vi "XY Sub_VI.vi"(3 "error in (no error)":errorcluster, 5 "XY Cluster In":T1 {"Y Data"."Input"."Tol" min=0.0; "X Data"."Input"."Tol" min=0.0}) -> (0 "error out":errorcluster, 2 "XY Cluster Out":T1={"X Data"={"Complete?"=FALSE, "Motor Params"={"Duty %"=0.0, "X Freq"=0.0, "FWD/RVS"=FALSE}, "SP"={"Accel"=0.0, "Decel"=0.0, "Speed"=0.0}, "State"=enum."Stop", "Input"={"Coord"=0.0, "Tol"=0.0, "Accel"=0.0, "Decel"=0.0, "Max Speed"=0.0}, "Path"={"V plan"=[], "V actual"=[], "S actual"=[], "a actual"=[], "Profile"=enum."Triangular", "Decel Dist"=0.0, "Accel Dist"=0.0, "Cruise V"=0.0, "Cruise Dist"=0.0}, "PID"={"Kc"=0.0, "Ti"=0.0, "Td"=0.0}, "Motion"={"Speed"=0.0, "Dist"=0.0, "Acceleration"=0.0, "Dist to target"=0.0}}, "Y Data"={"Complete?"=FALSE, "Motor Params"={"Duty %"=0.0, "Freq"=0.0, "FWD/RVS"=FALSE}, "SP"={"Y Accel"=0.0, "Y Decel"=0.0, "Speed"=0.0}, "State"=enum."Stop", "Input"={"Coord"=0.0, "Tol"=0.0, "Accel"=0.0, "Decel"=0.0, "Max Speed"=0.0}, "Path"={"V plan"=[], "V actual"=[], "S actual"=[], "a actual"=[], " Profile"=enum."Triangular", "Decel Dist"=0.0, "Accel Dist"=0.0, "Cruise V"=0.0, "Cruise Dist"=0.0}, "PID"={"Kc"=0.0, "Ti"=0.0, "Td"=0.0}, "Motion"={"Speed"=0.0, "Dist"=0.0, "Acceleration"=0.0, "Dist to target"=0.0}}, "Timing"={"Runtime"=0.0, "Loop time"=0.0, "Loop iter"=0, "Tick"=0.0}, "stop"=FALSE} {"Y Data"."Input"."Tol" min=0.0; "X Data"."Input"."Tol" min=0.0})   [LabVIEW 2017]
uses:
  Encoder Cluster.ctl
  <vilib>/myRIO/Common/Instrument Driver Framework/myRIO v1.0/Encoder/typedefs/Encoder Count Direction Enum.ctl
  XY Cluster.ctl
  Motor Status Enum.ctl
  Motion Type Def.ctl
  <vilib>/myRIO/Instrument Drivers/Onboard IO/PWM/typedefs/PWM Reference.ctl
  <vilib>/myRIO/Common/Instrument Driver Framework/Utilities/typedefs/myRIO Generic Hardware Reference.ctl
  <vilib>/myRIO/Common/Instrument Driver Framework/Utilities/typedefs/Hardware Version Enum.ctl
  <vilib>/myRIO/Common/Instrument Driver Framework/Utilities/typedefs/myRIO v1.0 Reference.ctl
  <vilib>/myRIO/Common/Instrument Driver Framework/Utilities/typedefs/Generic FPGA Reference.ctl
  <vilib>/myRIO/Common/Instrument Driver Framework/myRIO v1.0/PWM/typedefs/PWM Channels Enum.ctl
  <vilib>/myRIO/Instrument Drivers/Onboard IO/PWM/typedefs/PWM Configuration.ctl
  <vilib>/userdefined/High Color/nirio_resource_hc.ctl
  <vilib>/myRIO/Common/Instrument Driver Framework/Utilities/vis/Is FPGA Ref Available.vi
  <vilib>/myRIO/Common/Instrument Driver Framework/myRIO v1.0/PWM/vis/myRIO v1.1 Open PWM.vi
  <vilib>/myRIO/Instrument Drivers/Onboard IO/PWM/vis/Set Duty Cycle and Frequency.vi
  <vilib>/myRIO/Common/Instrument Driver Framework/Utilities/vis/Validate Channels.vi
  <vilib>/myRIO/Common/Instrument Driver Framework/myRIO v1.0/PWM/vis/myRIO v1.0 Reserve PWM.vi
  <vilib>/myRIO/Common/Instrument Driver Framework/myRIO v1.0/PWM/vis/myRIO v1.0 Build MUX Configuration PWM.vi
  <vilib>/myRIO/Common/Instrument Driver Framework/myRIO v1.0/Resource Manager/vis/myRIO v1.0 Reserve Channel List.vi
  <vilib>/myRIO/Common/Instrument Driver Framework/myRIO v1.0/Resource Manager/vis/myRIO v1.0 Create Configuration List.vi
  <vilib>/myRIO/Common/Instrument Driver Framework/myRIO v1.0/Resource Manager/vis/myRIO v1.0 Reserve Channel.vi
  <vilib>/myRIO/Common/Instrument Driver Framework/myRIO v1.0/Resource Manager/vis/myRIO v1.0 Unreserve Channel.vi
  <vilib>/myRIO/Common/Instrument Driver Framework/myRIO v1.0/Resource Manager/vis/myRIO v1.0 Build Mutex Name.vi
  <vilib>/addons/control/pid/pid.llb/PID Control Input Filter (DBL).vi
  <vilib>/addons/control/pid/pid.llb/PID (DBL).vi
  <vilib>/Utility/VariantDataType/GetNumericInfo.vi
  <vilib>/Utility/error.llb/Error Cluster From Error Code.vi
  <vilib>/myRIO/Common/Instrument Driver Framework/myRIO v1.0/myRIO v1.1 Open.vi
  <vilib>/myRIO/Common/Instrument Driver Framework/Utilities/vis/IO Manager.vi
  <vilib>/myRIO/Common/Instrument Driver Framework/Utilities/vis/Configuration Manager.vi
  <vilib>/myRIO/Common/Instrument Driver Framework/myRIO v1.0/Resource Manager/vis/myRIO v1.0 Configure IO.vi
  <vilib>/myRIO/Common/Instrument Driver Framework/myRIO v1.0/myRIO v1.0 Close.vi
  <vilib>/myRIO/Common/Instrument Driver Framework/myRIO v1.0/PWM/vis/myRIO v1.0 Write PWM.vi
  <vilib>/myRIO/Express VI/Onboard IO/PWM/PWM Express VI.xnode
  <vilib>/myRIO/Instrument Drivers/Onboard IO/PWM/vis/myRIO PWM Open.xnode
  <vilib>/addons/control/pid/NI_PID_pid.lvlib
  <vilib>/ptbypt/NI_PtbyPt.lvlib
  <vilib>/myRIO/Instrument Drivers/Onboard IO/PWM/PWM.lvlib
panel:
  out "Y PID":cluster{"mean":dbl, "output":dbl}(graph)
  out "X PID":cluster{"Speed":dbl, "output":dbl}(graph)
  out "Y dist > +20":bool
  out "X dist > +20":bool
  out "Encoder Output":T4
  out "X&Y Complete":bool
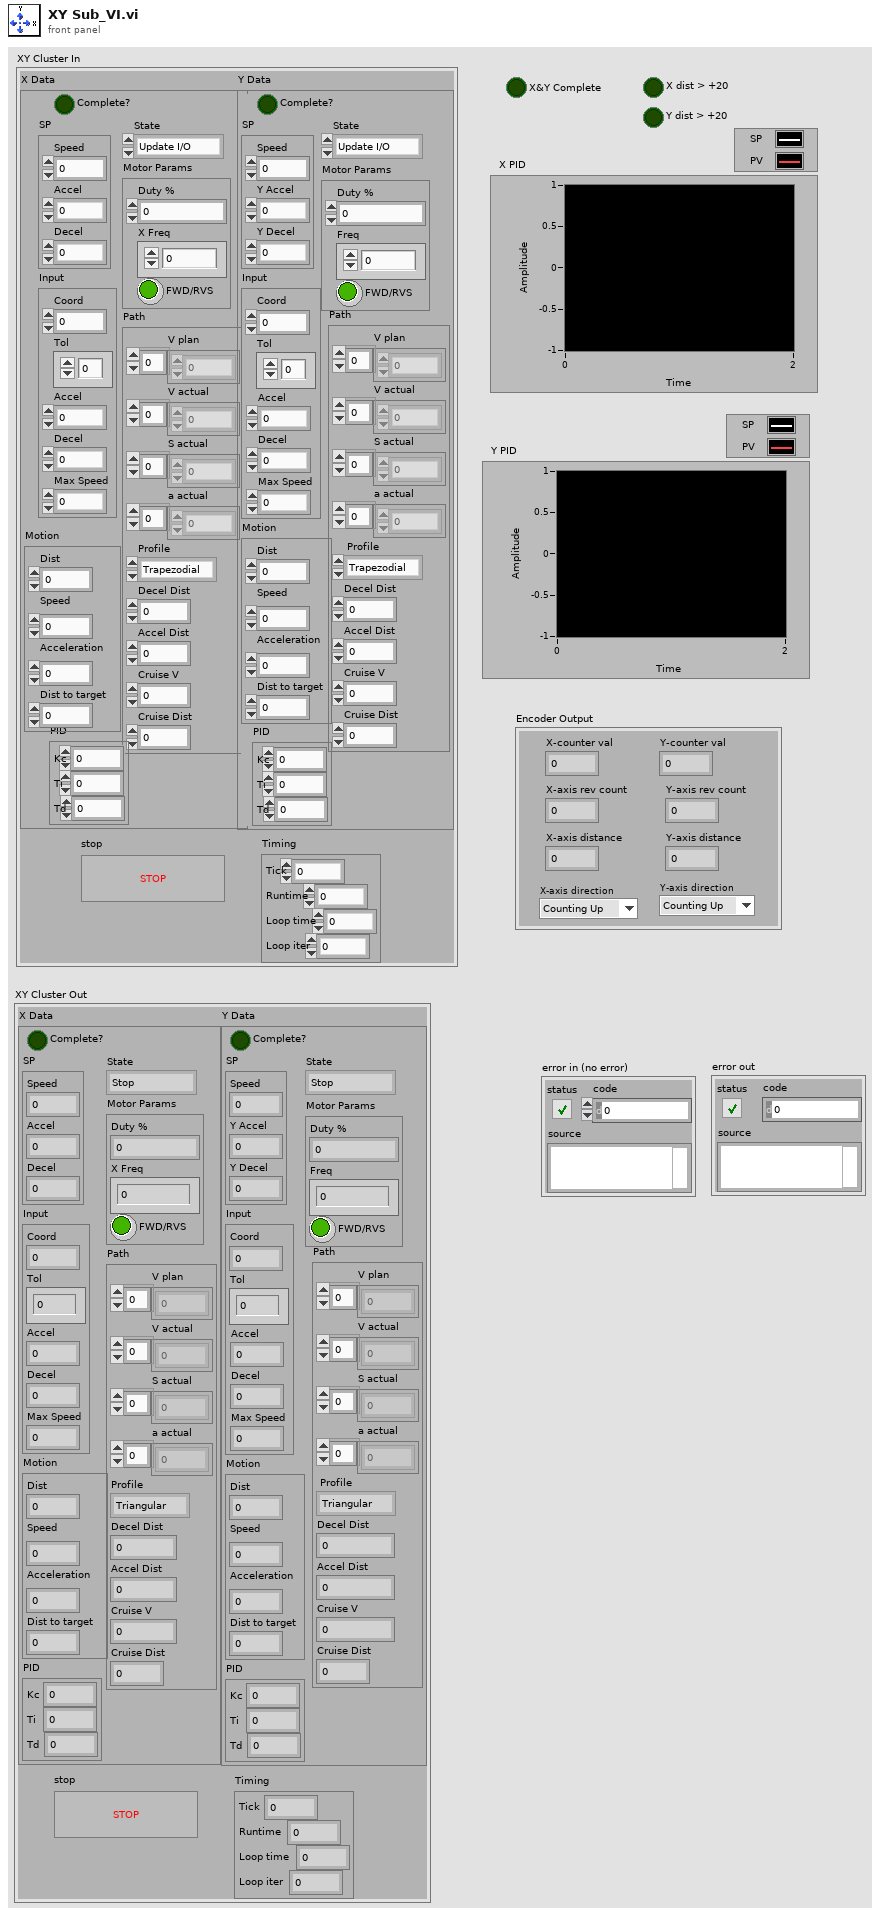
[diagram p1: front panel]
types:
  T1 = typedef "XY Cluster.ctl" = cluster{"X Data":cluster{"Complete?":bool, "Motor Params":cluster{"Duty %":dbl, "X Freq":dbl, "FWD/RVS":bool}, "SP":cluster{"Accel":dbl, "Decel":dbl, "Speed":dbl}, "State":T2, "Input":cluster{"Coord":dbl, "Tol":dbl, "Accel":dbl, "Decel":dbl, "Max Speed":dbl}, "Path":cluster{"V plan":dbl[], "V actual":dbl[], "S actual":dbl[], "a actual":dbl[], "Profile":T3, "Decel Dist":dbl, "Accel Dist":dbl, "Cruise V":dbl, "Cruise Dist":dbl}, "PID":cluster{"Kc":dbl, "Ti":dbl, "Td":dbl}, "Motion":cluster{"Speed":dbl, "Dist":dbl, "Acceleration":dbl, "Dist to target":dbl}}, "Y Data":cluster{"Complete?":bool, "Motor Params":cluster{"Duty %":dbl, "Freq":dbl, "FWD/RVS":bool}, "SP":cluster{"Y Accel":dbl, "Y Decel":dbl, "Speed":dbl}, "State":T2, "Input":cluster{"Coord":dbl, "Tol":dbl, "Accel":dbl, "Decel":dbl, "Max Speed":dbl}, "Path":cluster{"V plan":dbl[], "V actual":dbl[], "S actual":dbl[], "a actual":dbl[], " Profile":T3, "Decel Dist":dbl, "Accel Dist":dbl, "Cruise V":dbl, "Cruise Dist":dbl}, "PID":cluster{"Kc":dbl, "Ti":dbl, "Td":dbl}, "Motion":cluster{"Speed":dbl, "Dist":dbl, "Acceleration":dbl, "Dist to target":dbl}}, "Timing":cluster{"Runtime":dbl, "Loop time":dbl, "Loop iter":i32, "Tick":dbl}, "stop":bool}
  T2 = typedef "Motor Status Enum.ctl" = enum16{"Update I/O", "Stop", "Steady Speed", "Accelerate", "Decelerate", "Drive Motor"}
  T3 = typedef "Motion Type Def.ctl" = enum16{"Trapezodial", "Triangular"}
  T4 = typedef "Encoder Cluster.ctl" = cluster{"Y-axis rev count":dbl, "Y-axis distance":dbl, "X-axis rev count":dbl, "X-axis distance":dbl, "Y-axis direction":T5, "X-axis direction":T5, "X-counter val":i32, "Y-counter val":i32}
  T5 = typedef "Encoder Count Direction Enum.ctl" = enum16{"Counting Up", "Counting Down"}
  T6 = cluster{"X Axis":cluster{"Displacement":dbl, "Speed SP":dbl, "Speed PV":dbl, "Acceleration":dbl}, "Y Axis":cluster{"Displacement":dbl, "Speed SP":dbl, "Speed PV":dbl, "Acceleration":dbl}, "XY Complete?":bool}
  T7 = cluster{" Distance target (mm)":dbl, "Max Accel (mm/s^2)":dbl, "Max Decel (mm/s^2)":dbl, "Velocity Limit (mm/s) ":dbl}
  T8 = cluster{"Complete?":bool, "Motor Params":cluster{"Duty %":dbl, "X Freq":dbl, "FWD/RVS":bool}, "SP":cluster{"Accel":dbl, "Decel":dbl, "Speed":dbl}, "State":T2, "Input":cluster{"Coord":dbl, "Tol":dbl, "Accel":dbl, "Decel":dbl, "Max Speed":dbl}, "Path":cluster{"V plan":dbl[], "V actual":dbl[], "S actual":dbl[], "a actual":dbl[], "Profile":T3, "Decel Dist":dbl, "Accel Dist":dbl, "Cruise V":dbl, "Cruise Dist":dbl}, "PID":cluster{"Kc":dbl, "Ti":dbl, "Td":dbl}, "Motion":cluster{"Speed":dbl, "Dist":dbl, "Acceleration":dbl, "Dist to target":dbl}}
  T9 = cluster{"Crusing Time (s)":dbl, "Decel Time (s)":dbl, "Accel Time (s)":dbl, "Total Time (s)":dbl, "Accel Distance (mm)":dbl, "Decel Distance (mm)":dbl, "Crusing Distance (mm)":dbl, "Total Dist (mm)":dbl, "Max Speed (mm/s)":dbl}
  T10 = cluster{"Complete?":bool, "Motor Params":cluster{"Duty %":dbl, "Freq":dbl, "FWD/RVS":bool}, "SP":cluster{"Y Accel":dbl, "Y Decel":dbl, "Speed":dbl}, "State":T2, "Input":cluster{"Coord":dbl, "Tol":dbl, "Accel":dbl, "Decel":dbl, "Max Speed":dbl}, "Path":cluster{"V plan":dbl[], "V actual":dbl[], "S actual":dbl[], "a actual":dbl[], " Profile":T3, "Decel Dist":dbl, "Accel Dist":dbl, "Cruise V":dbl, "Cruise Dist":dbl}, "PID":cluster{"Kc":dbl, "Ti":dbl, "Td":dbl}, "Motion":cluster{"Speed":dbl, "Dist":dbl, "Acceleration":dbl, "Dist to target":dbl}}
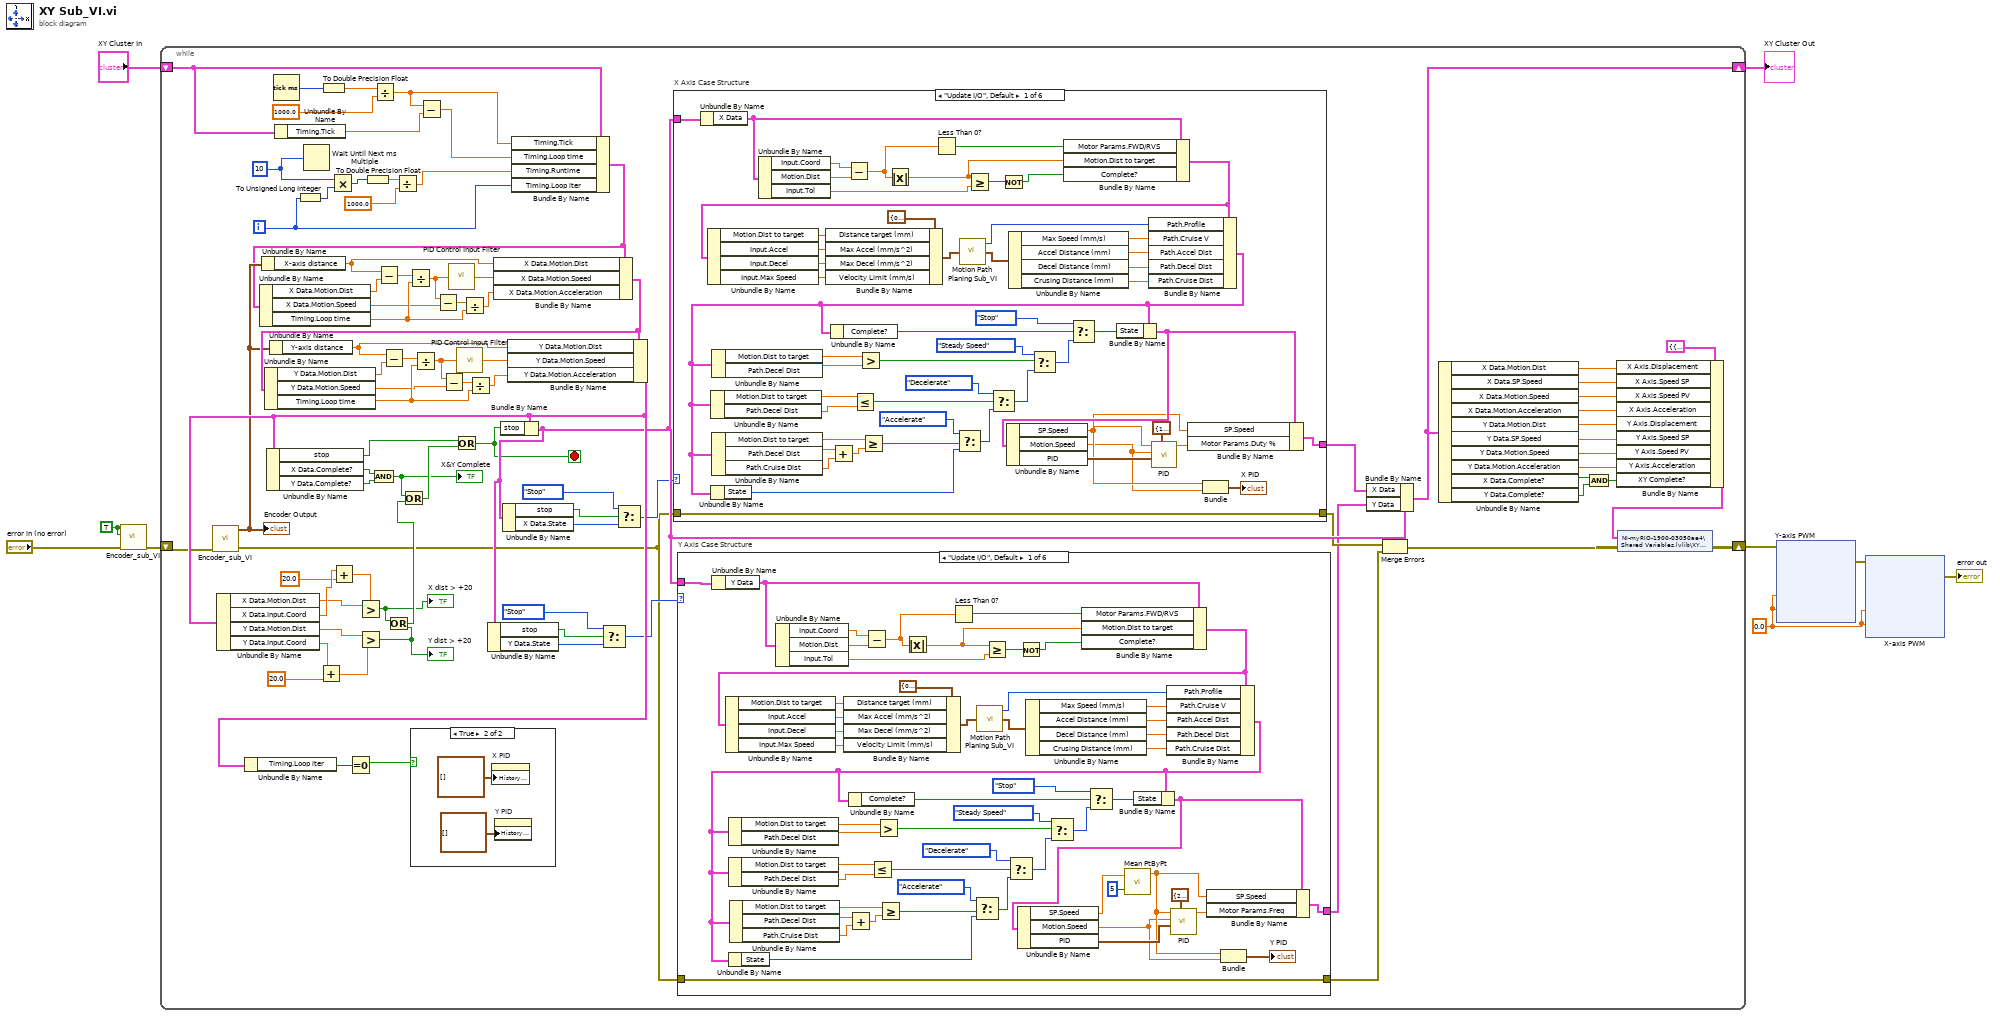
[diagram p0: block diagram]
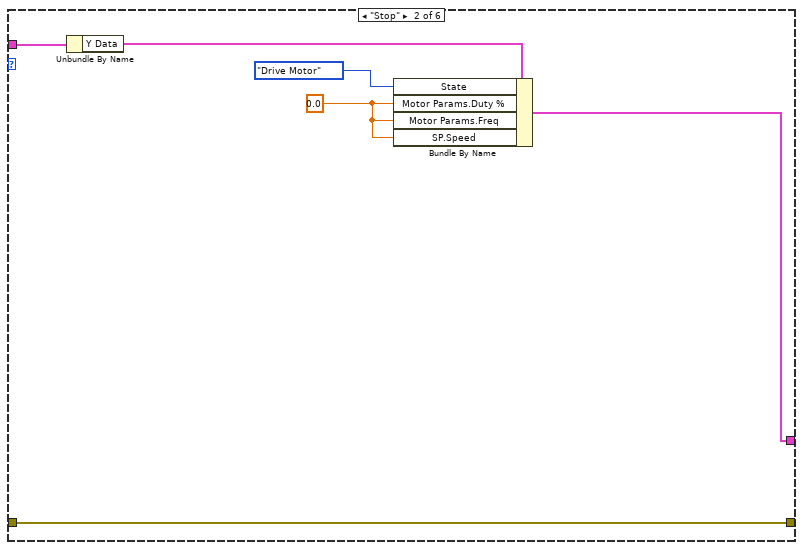
[diagram p3: hidden frame]
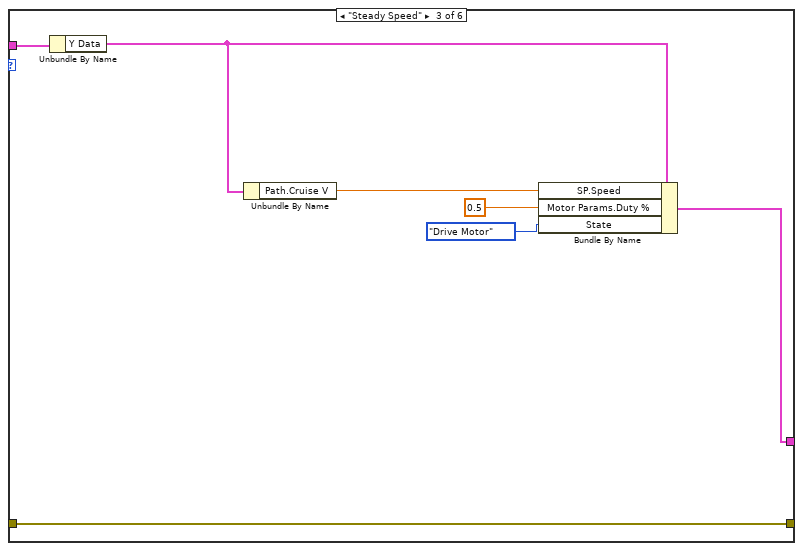
[diagram p4: hidden frame]
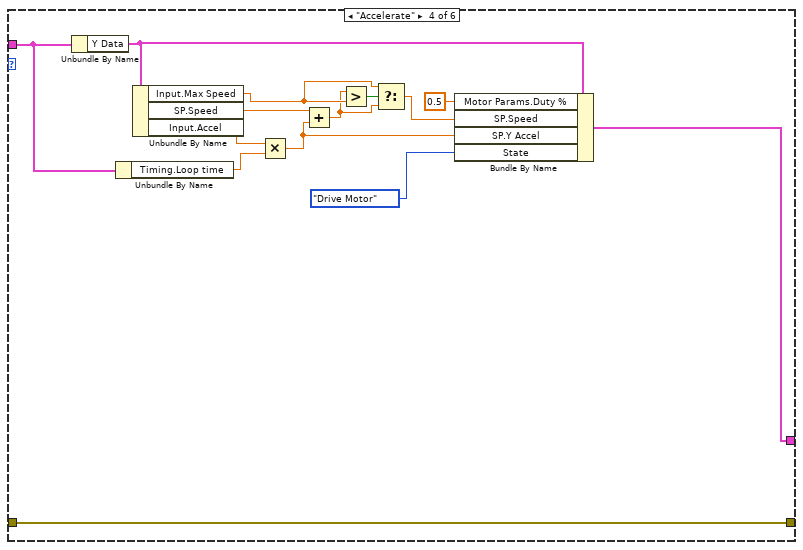
[diagram p5: hidden frame]
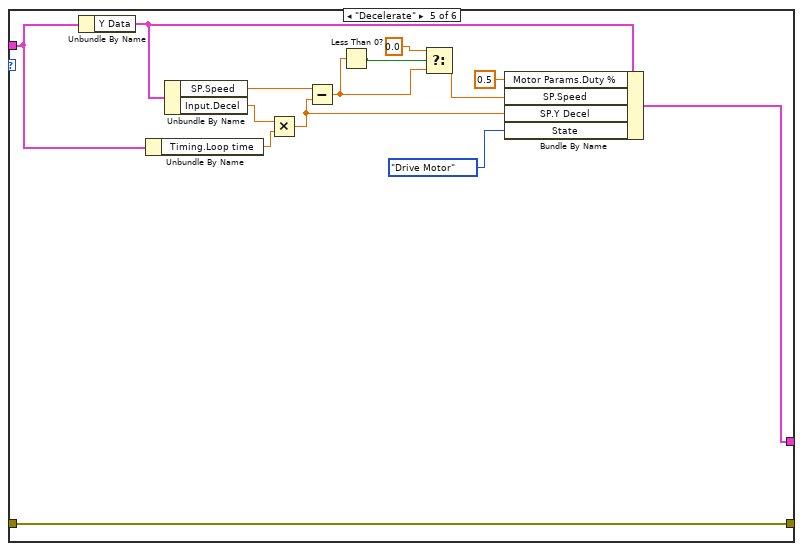
[diagram p6: hidden frame]
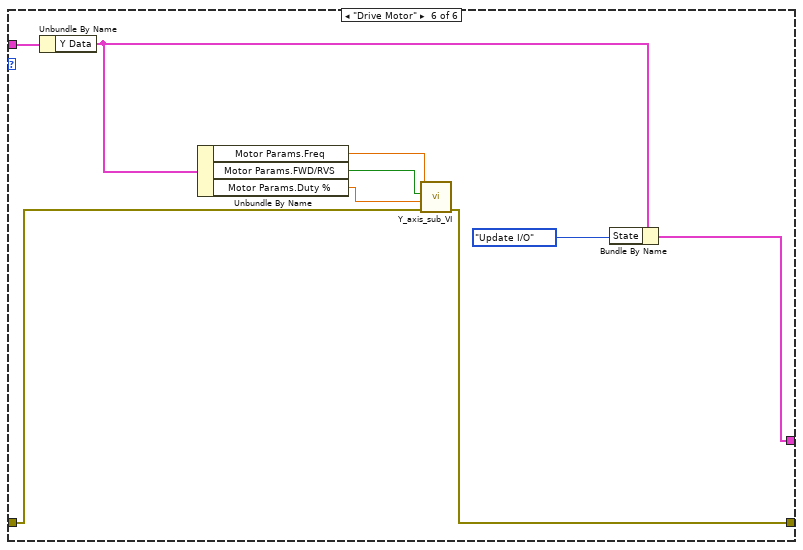
[diagram p7: hidden frame]
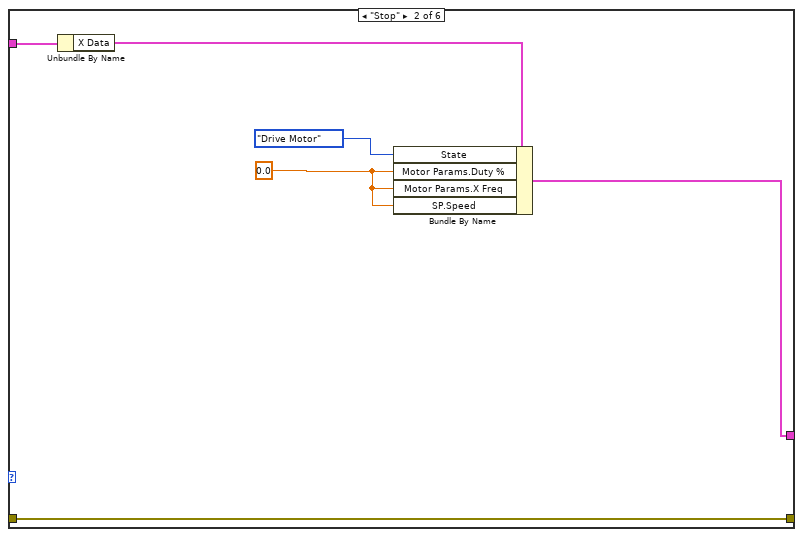
[diagram p8: hidden frame]
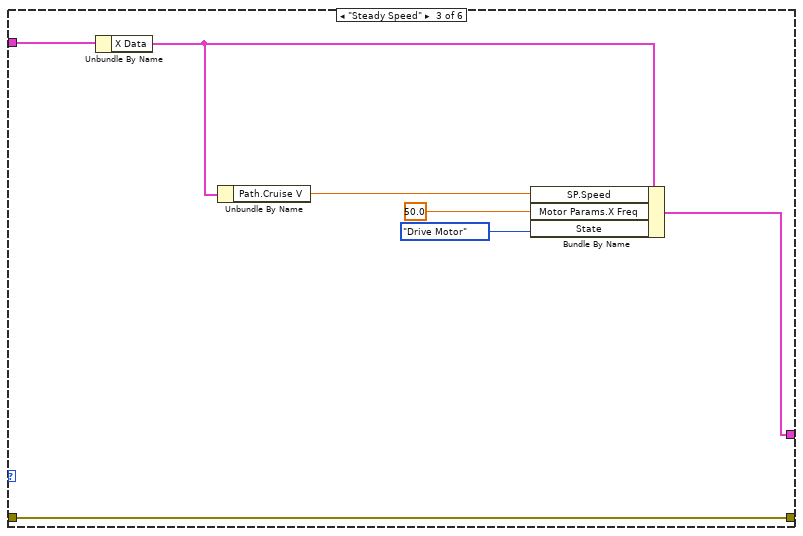
[diagram p9: hidden frame]
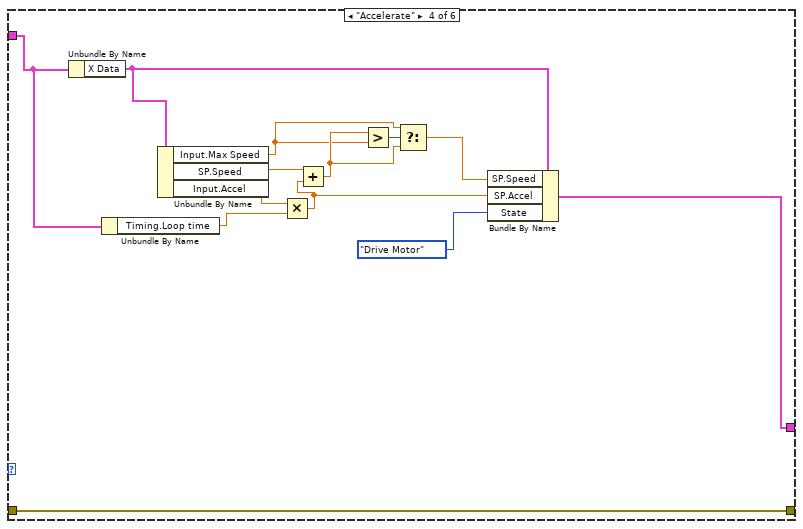
[diagram p10: hidden frame]
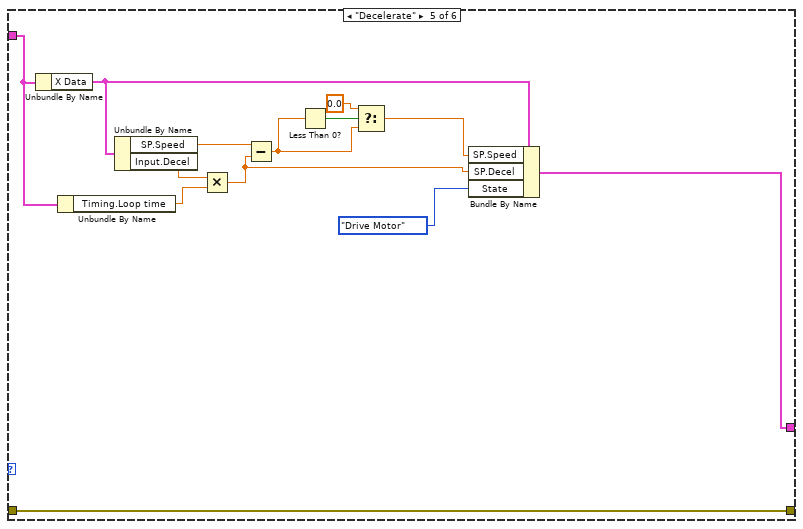
[diagram p11: hidden frame]
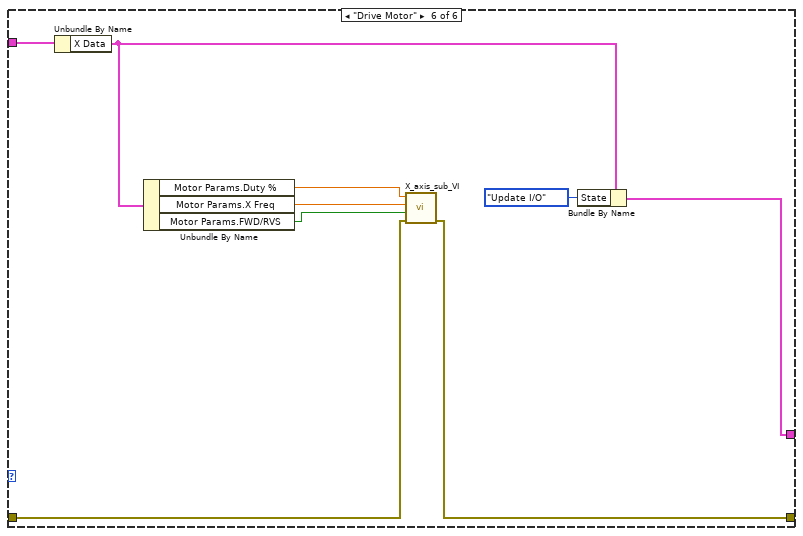
[diagram p12: hidden frame]
diagram:
  w3 = 0.0 ("Frequency [Hz]")
  w8 = TRUE ("Reset X Counter")
  n1 = call "Encoder_sub_VI.vi"("error in (no error)"="error in (no error)", "Reset Y Counter"=w8, "Reset X Counter"=w8) -> ("error out"=w6:errorcluster)  [unwired: 7 in, 1 out]
  n2 = while {
    shift-right: [w28] -> w5
    shift-left: "XY Cluster In" -> [w31]
    shift-right: [w18] -> w2
    shift-left: w6 -> [w34]
    i -> [w33]
    stop <- w32 stop-if-true
    w46 = u32 10 ("millisecond multiple")
    n3 = call "Encoder_sub_VI.vi"("error in (no error)"=w34) -> ("error out"=w65:errorcluster, "Encoder Output"=w56:T4)  [unwired: 9 in]
    "Encoder Output" <- w56
    n4 = Unbundle By Name(w56) -> ("X-axis distance"=w49:dbl)
    n5 = Unbundle By Name(w56) -> ("Y-axis distance"=w64:dbl)
    n6 = Tick Count (ms)() -> (millisecond timer value=w40:u32)
    n7 = Unbundle By Name(w31) -> ("Timing.Tick"=w37:dbl)
    n8 = To Unsigned Long Integer(number=w33) -> (unsigned 32bit integer=w45:u32)
    n9 = Wait Until Next ms Multiple(millisecond multiple=w46) -> ()  [unwired: 1 out]
    n10 = To Double Precision Float(number=w40) -> (double precision float=w38:dbl)
    n11 = Multiply(x=w46, y=w45) -> (x*y=w44:u32)
    n12 = To Double Precision Float(number=w44) -> (double precision float=w42:dbl)
    n13 = Divide(x=w38, y=1000.0) -> (x/y=w36:dbl)
    n14 = Divide(x=w42, y=1000.0) -> (x/y=w41:dbl)
    n15 = Subtract(x=w36, y=w37) -> (x-y=w35:dbl)
    n16 = Bundle By Name(cluster=w31, "Timing.Tick"=w36, "Timing.Loop time"=w35, "Timing.Runtime"=w41, "Timing.Loop iter"=w33) -> (w30:T1)
    n17 = Unbundle By Name(w30) -> ("X Data.Motion.Dist"=w50:dbl, "X Data.Motion.Speed"=w53:dbl, "Timing.Loop time"=w54:dbl)
    n18 = Subtract(x=w49, y=w50) -> (x-y=w51:dbl)
    n19 = Divide(x=w51, y=w54) -> (x/y=w13:dbl)
    n20 = Subtract(x=w13, y=w53) -> (x-y=w52:dbl)
    n21 = call-poly <vilib>:"PID Control Input Filter.vi"("input"=w13) -> ("output"=w12:dbl)  [unwired: 4 in]
    n22 = Divide(x=w52, y=w54) -> (x/y=w55:dbl)
    n23 = Bundle By Name(cluster=w30, "X Data.Motion.Dist"=w49, "X Data.Motion.Speed"=w12, "X Data.Motion.Acceleration"=w55) -> (w63:T1)
    n24 = Unbundle By Name(w63) -> ("Y Data.Motion.Dist"=w57:dbl, "Y Data.Motion.Speed"=w60:dbl, "Timing.Loop time"=w61:dbl)
    n25 = Subtract(x=w64, y=w57) -> (x-y=w58:dbl)
    n26 = Divide(x=w58, y=w61) -> (x/y=w11:dbl)
    n27 = Subtract(x=w11, y=w60) -> (x-y=w59:dbl)
    n28 = call-poly <vilib>:"PID Control Input Filter.vi"("input"=w11) -> ("output"=w10:dbl)  [unwired: 4 in]
    n29 = Divide(x=w59, y=w61) -> (x/y=w62:dbl)
    n30 = Bundle By Name(cluster=w63, "Y Data.Motion.Dist"=w64, "Y Data.Motion.Speed"=w10, "Y Data.Motion.Acceleration"=w62) -> (w92:T1)
    n31 = Unbundle By Name(w92) -> ("X Data.Motion.Dist"=w80:dbl, "X Data.Input.Coord"=w87:dbl, "Y Data.Motion.Dist"=w82:dbl, "Y Data.Input.Coord"=w90:dbl)
    n32 = Unbundle By Name(w92) -> ("Timing.Loop iter"=w94:i32)
    n33 = Unbundle By Name(w92) -> ("stop"=w47:bool, "X Data.Complete?"=w77:bool, "Y Data.Complete?"=w78:bool)
    n34 = Add(x=w90, y=20.0) -> (x+y=w91:dbl)
    n35 = Add(x=w87, y=20.0) -> (x+y=w88:dbl)
    n36 = Equal To 0?(x=w94) -> (x = 0?=w93:bool)
    n37 = Greater?(x=w80, y=w88) -> (0:w81:bool)
    "X dist > +20" <- w81
    n38 = Greater?(x=w82, y=w91) -> (0:w85:bool)
    "Y dist > +20" <- w85
    n39 = And(x=w77, y=w78) -> (x .and. y?=w84:bool)
    "X&Y Complete" <- w84
    n40 = Or(x=w81, y=w85) -> (x .or. y?=w83:bool)
    n41 = Or(x=w84, y=w83) -> (x .or. y?=w95:bool)
    n42 = case shown="True" w93 {
      frame False {
      }
      frame True {
        n43 = property on="X PID" class="WFChart (strict)"("History Data"=cluster{"Speed":dbl, "output":dbl}[] []) -> ()  [unwired: 2 in, 2 out]
        n44 = property on="Y PID" class="WFChart (strict)"("History Data"=cluster{"mean":dbl, "output":dbl}[] []) -> ()  [unwired: 2 in, 2 out]
      }
    }
    n45 = Or(x=w47, y=w95) -> (x .or. y?=w32:bool)
    n46 = Bundle By Name(cluster=w92, "stop"=w32) -> (w79:T1)
    n47 = Unbundle By Name(w79) -> ("stop"=w74:bool, "Y Data.State"=w73:T2)
    n48 = Unbundle By Name(w79) -> ("stop"=w70:bool, "X Data.State"=w69:T2)
    n49 = Select(t=Motor_Status_Enum."Stop", s=w74, f=w73) -> (s? t:f=w76:T2)
    n50 = Select(t=Motor_Status_Enum."Stop", s=w70, f=w69) -> (s? t:f=w72:T2)
    n51 = case "X Axis Case Structure" shown="\"Update I/O\", Default" w72 {
      tunnel: [w229 w263 w268 w282 w290 w298] -> w48
      tunnel: w65 -> [w249 w259 w266 w280 w289 w301]
      tunnel: [w249 w259 w266 w280 w289 w300] -> w67
      tunnel: w79 -> [w230 w261 w269 w281 w292 w305]
      frame "Update I/O", Default {
        n52 = Unbundle By Name(w230) -> ("X Data"=w212:T8)
        n53 = Unbundle By Name(w212) -> ("Input.Coord"=w257:dbl, "Motion.Dist"=w252:dbl, "Input.Tol"=w256:dbl)
        n54 = Subtract(x=w257, y=w252) -> (x-y=w253:dbl)
        n55 = Absolute Value(x=w253) -> (abs(x)=w227:dbl)
        n56 = Less Than 0?(x=w253) -> (x < 0?=w228:bool)
        n57 = Greater Or Equal?(x=w227, y=w256) -> (x >= y?=w255:bool)
        n58 = Not(x=w255) -> (.not. x?=w254:bool)
        n59 = Bundle By Name(cluster=w212, "Motor Params.FWD/RVS"=w228, "Motion.Dist to target"=w227, "Complete?"=w254) -> (w225:T8)
        n60 = Unbundle By Name(w225) -> ("Motion.Dist to target"=w226:dbl, "Input.Accel"=w246:dbl, "Input.Decel"=w245:dbl, "Input.Max Speed"=w247:dbl)
        n61 = Bundle By Name(cluster=T7 {" Distance target (mm)"=0.0, "Max Accel (mm/s^2)"=0.0, "Max Decel (mm/s^2)"=0.0, "Velocity Limit (mm/s) "=0.0} ("Motion Planning Inputs"), "Distance target (mm)"=w226, "Max Accel (mm/s^2)"=w246, "Max Decel (mm/s^2)"=w245, "Velocity Limit (mm/s)"=w247) -> (w209:T7)
        n62 = call "Motion Path Planing Sub_VI.vi"("Motion Planning Inputs"=w209) -> ("Motion Profile"=w208:T3, "Motion Planning Outputs"=w207:T9)  [unwired: 5 in]
        n63 = Unbundle By Name(w207) -> ("Max Speed (mm/s)"=w248:dbl, "Accel Distance (mm)"=w244:dbl, "Decel Distance (mm)"=w243:dbl, "Crusing Distance (mm)"=w224:dbl)
        n64 = Bundle By Name(cluster=w225, "Path.Profile"=w208, "Path.Cruise V"=w248, "Path.Accel Dist"=w244, "Path.Decel Dist"=w243, "Path.Cruise Dist"=w224) -> (w219:T8)
        n65 = Unbundle By Name(w219) -> ("Motion.Dist to target"=w221:dbl, "Path.Decel Dist"=w220:dbl)
        n66 = Unbundle By Name(w219) -> ("State"=w241:T2)
        n67 = Unbundle By Name(w219) -> ("Motion.Dist to target"=w223:dbl, "Path.Decel Dist"=w222:dbl)
        n68 = Unbundle By Name(w219) -> ("Motion.Dist to target"=w215:dbl, "Path.Decel Dist"=w218:dbl, "Path.Cruise Dist"=w217:dbl)
        n69 = Unbundle By Name(w219) -> ("Complete?"=w233:bool)
        n70 = Add(x=w218, y=w217) -> (x+y=w216:dbl)
        n71 = Less Or Equal?(x=w221, y=w220) -> (x <= y?=w240:bool)
        n72 = Greater?(x=w223, y=w222) -> (0:w236:bool)
        n73 = Greater Or Equal?(x=w215, y=w216) -> (x >= y?=w214:bool)
        n74 = Select(t=Motor_Status_Enum."Accelerate" ("State"), s=w214, f=w241) -> (s? t:f=w239:T2)
        n75 = Select(t=Motor_Status_Enum."Decelerate" ("State"), s=w240, f=w239) -> (s? t:f=w235:T2)
        n76 = Select(t=Motor_Status_Enum."Steady Speed" ("State"), s=w236, f=w235) -> (s? t:f=w234:T2)
        n77 = Select(t=Motor_Status_Enum."Stop" ("State"), s=w233, f=w234) -> (s? t:f=w231:T2)
        n78 = Bundle By Name(cluster=w219, "State"=w231) -> (w213:T8)
        n79 = Unbundle By Name(w213) -> ("SP.Speed"=w205:dbl, "Motion.Speed"=w204:dbl, "PID"=w251:cluster{"Kc":dbl, "Ti":dbl, "Td":dbl})
        n80 = call-poly <vilib>:"PID.vi"("output range"=cluster{"output high":dbl, "output low":dbl} {"output high"=100.0, "output low"=0.0}, "PID gains"=w251, "process variable"=w204, "setpoint"=w205) -> ("output"=w211:dbl)  [unwired: 6 in, 1 out]
        n81 = Bundle By Name(cluster=w213, "SP.Speed"=w205, "Motor Params.Duty %"=w211) -> (w229:T8)
        n82 = Bundle("Speed"=w205, "Speed"=w204) -> (→"X PID":cluster{"Speed":dbl, "Speed":dbl})  [unwired: 1 in]
      }
      frame "Stop" {
        w258 = 0.0
        n83 = Unbundle By Name(w261) -> ("X Data"=w260:T8)
        n84 = Bundle By Name(cluster=w260, "State"=Motor_Status_Enum."Drive Motor", "Motor Params.Duty %"=w258, "Motor Params.X Freq"=w258, "SP.Speed"=w258) -> (w263:T8)
      }
      frame "Steady Speed" {
        n85 = Unbundle By Name(w269) -> ("X Data"=w265:T8)
        n86 = Unbundle By Name(w265) -> ("Path.Cruise V"=w264:dbl)
        n87 = Bundle By Name(cluster=w265, "SP.Speed"=w264, "Motor Params.X Freq"=50.0 ("Motor Params.Duty %"), "State"=Motor_Status_Enum."Drive Motor") -> (w268:T8)
      }
      frame "Accelerate" {
        n88 = Unbundle By Name(w281) -> ("X Data"=w283:T8)
        n89 = Unbundle By Name(w281) -> ("Timing.Loop time"=w279:dbl)
        n90 = Unbundle By Name(w283) -> ("Input.Max Speed"=w271:dbl, "SP.Speed"=w277:dbl, "Input.Accel"=w276:dbl)
        n91 = Multiply(x=w276, y=w279) -> (x*y=w275:dbl)
        n92 = Add(x=w277, y=w275) -> (x+y=w272:dbl)
        n93 = Greater?(x=w272, y=w271) -> (0:w274:bool)
        n94 = Select(t=w271, s=w274, f=w272) -> (s? t:f=w273:dbl)
        n95 = Bundle By Name(cluster=w283, "SP.Speed"=w273, "SP.Accel"=w275, "State"=Motor_Status_Enum."Drive Motor") -> (w282:T8)
      }
      frame "Decelerate" {
        n96 = Unbundle By Name(w292) -> ("X Data"=w291:T8)
        n97 = Unbundle By Name(w292) -> ("Timing.Loop time"=w296:dbl)
        n98 = Unbundle By Name(w291) -> ("SP.Speed"=w294:dbl, "Input.Decel"=w293:dbl)
        n99 = Multiply(x=w293, y=w296) -> (x*y=w288:dbl)
        n100 = Subtract(x=w294, y=w288) -> (x-y=w284:dbl)
        n101 = Less Than 0?(x=w284) -> (x < 0?=w287:bool)
        n102 = Select(t=0.0, s=w287, f=w284) -> (s? t:f=w286:dbl)
        n103 = Bundle By Name(cluster=w291, "SP.Speed"=w286, "SP.Decel"=w288, "State"=Motor_Status_Enum."Drive Motor") -> (w290:T8)
      }
      frame "Drive Motor" {
        n104 = Unbundle By Name(w305) -> ("X Data"=w299:T8)
        n105 = Unbundle By Name(w299) -> ("Motor Params.Duty %"=w304:dbl, "Motor Params.X Freq"=w303:dbl, "Motor Params.FWD/RVS"=w302:bool)
        n106 = call "X_axis_sub_VI.vi"("error in (no error)"=w301, "FWD/RVS"=w302, "Frequency"=w303, "Duty Cycle %"=w304) -> ("error out"=w300:errorcluster)  [unwired: 7 in]
        n107 = Bundle By Name(cluster=w299, "State"=Motor_Status_Enum."Update I/O") -> (w298:T8)
      }
    }
    n108 = case "Y Axis Case Structure" shown="\"Update I/O\", Default" w76 {
      tunnel: [w109 w159 w164 w179 w189 w197] -> w66
      tunnel: w65 -> [w153 w155 w163 w177 w188 w203]
      tunnel: [w153 w155 w163 w177 w188 w202] -> w68
      tunnel: w79 -> [w152 w157 w165 w178 w191 w201]
      frame "Update I/O", Default {
        n109 = Unbundle By Name(w152) -> ("Y Data"=w108:T10)
        n110 = Unbundle By Name(w108) -> ("Input.Coord"=w151:dbl, "Motion.Dist"=w147:dbl, "Input.Tol"=w150:dbl)
        n111 = Subtract(x=w151, y=w147) -> (x-y=w112:dbl)
        n112 = Absolute Value(x=w112) -> (abs(x)=w125:dbl)
        n113 = Less Than 0?(x=w112) -> (x < 0?=w111:bool)
        n114 = Greater Or Equal?(x=w125, y=w150) -> (x >= y?=w149:bool)
        n115 = Not(x=w149) -> (.not. x?=w148:bool)
        n116 = Bundle By Name(cluster=w108, "Motor Params.FWD/RVS"=w111, "Motion.Dist to target"=w125, "Complete?"=w148) -> (w123:T10)
        n117 = Unbundle By Name(w123) -> ("Motion.Dist to target"=w124:dbl, "Input.Accel"=w141:dbl, "Input.Decel"=w140:dbl, "Input.Max Speed"=w142:dbl)
        n118 = Bundle By Name(cluster=T7 {" Distance target (mm)"=0.0, "Max Accel (mm/s^2)"=0.0, "Max Decel (mm/s^2)"=0.0, "Velocity Limit (mm/s) "=0.0} ("Motion Planning Inputs"), "Distance target (mm)"=w124, "Max Accel (mm/s^2)"=w141, "Max Decel (mm/s^2)"=w140, "Velocity Limit (mm/s)"=w142) -> (w103:T7)
        n119 = call "Motion Path Planing Sub_VI.vi"("Motion Planning Inputs"=w103) -> ("Motion Profile"=w102:T3, "Motion Planning Outputs"=w101:T9)  [unwired: 5 in]
        n120 = Unbundle By Name(w101) -> ("Max Speed (mm/s)"=w143:dbl, "Accel Distance (mm)"=w139:dbl, "Decel Distance (mm)"=w138:dbl, "Crusing Distance (mm)"=w122:dbl)
        n121 = Bundle By Name(cluster=w123, "Path.Profile"=w102, "Path.Cruise V"=w143, "Path.Accel Dist"=w139, "Path.Decel Dist"=w138, "Path.Cruise Dist"=w122) -> (w110:T10)
        n122 = Unbundle By Name(w110) -> ("Motion.Dist to target"=w121:dbl, "Path.Decel Dist"=w120:dbl)
        n123 = Unbundle By Name(w110) -> ("Motion.Dist to target"=w119:dbl, "Path.Decel Dist"=w118:dbl)
        n124 = Unbundle By Name(w110) -> ("State"=w136:T2)
        n125 = Unbundle By Name(w110) -> ("Motion.Dist to target"=w114:dbl, "Path.Decel Dist"=w117:dbl, "Path.Cruise Dist"=w116:dbl)
        n126 = Unbundle By Name(w110) -> ("Complete?"=w128:bool)
        n127 = Add(x=w117, y=w116) -> (x+y=w115:dbl)
        n128 = Less Or Equal?(x=w119, y=w118) -> (x <= y?=w135:bool)
        n129 = Greater?(x=w121, y=w120) -> (0:w131:bool)
        n130 = Greater Or Equal?(x=w114, y=w115) -> (x >= y?=w113:bool)
        n131 = Select(t=Motor_Status_Enum."Accelerate" ("State"), s=w113, f=w136) -> (s? t:f=w134:T2)
        n132 = Select(t=Motor_Status_Enum."Decelerate" ("State"), s=w135, f=w134) -> (s? t:f=w130:T2)
        n133 = Select(t=Motor_Status_Enum."Steady Speed" ("State"), s=w131, f=w130) -> (s? t:f=w129:T2)
        n134 = Select(t=Motor_Status_Enum."Stop" ("State"), s=w128, f=w129) -> (s? t:f=w126:T2)
        n135 = Bundle By Name(cluster=w110, "State"=w126) -> (w107:T10)
        n136 = Unbundle By Name(w107) -> ("SP.Speed"=w106:dbl, "Motion.Speed"=w98:dbl, "PID"=w146:cluster{"Kc":dbl, "Ti":dbl, "Td":dbl})
        n137 = call <vilib>:"Mean PtByPt.vi"("x"=w106, "sample length"=5) -> ("mean"=w99:dbl)  [unwired: 2 in, 1 out]
        n138 = call-poly <vilib>:"PID.vi"("output range"=cluster{"output high":dbl, "output low":dbl} {"output high"=23000.0, "output low"=0.0}, "PID gains"=w146, "process variable"=w98, "setpoint"=w99) -> ("output"=w144:dbl)  [unwired: 6 in, 1 out]
        n139 = Bundle By Name(cluster=w107, "SP.Speed"=w99, "Motor Params.Freq"=w144) -> (w109:T10)
        n140 = Bundle("mean"=w99, "Speed"=w98) -> (→"Y PID":cluster{"mean":dbl, "Speed":dbl})  [unwired: 1 in]
      }
      frame "Stop" {
        w154 = 0.0
        n141 = Unbundle By Name(w157) -> ("Y Data"=w156:T10)
        n142 = Bundle By Name(cluster=w156, "State"=Motor_Status_Enum."Drive Motor", "Motor Params.Duty %"=w154, "Motor Params.Freq"=w154, "SP.Speed"=w154) -> (w159:T10)
      }
      frame "Steady Speed" {
        n143 = Unbundle By Name(w165) -> ("Y Data"=w161:T10)
        n144 = Unbundle By Name(w161) -> ("Path.Cruise V"=w160:dbl)
        n145 = Bundle By Name(cluster=w161, "SP.Speed"=w160, "Motor Params.Duty %"=0.5, "State"=Motor_Status_Enum."Drive Motor") -> (w164:T10)
      }
      frame "Accelerate" {
        n146 = Unbundle By Name(w178) -> ("Y Data"=w180:T10)
        n147 = Unbundle By Name(w178) -> ("Timing.Loop time"=w176:dbl)
        n148 = Unbundle By Name(w180) -> ("Input.Max Speed"=w168:dbl, "SP.Speed"=w174:dbl, "Input.Accel"=w173:dbl)
        n149 = Multiply(x=w173, y=w176) -> (x*y=w172:dbl)
        n150 = Add(x=w174, y=w172) -> (x+y=w167:dbl)
        n151 = Greater?(x=w167, y=w168) -> (0:w170:bool)
        n152 = Select(t=w168, s=w170, f=w167) -> (s? t:f=w169:dbl)
        n153 = Bundle By Name(cluster=w180, "Motor Params.Duty %"=0.5, "SP.Speed"=w169, "SP.Y Accel"=w172, "State"=Motor_Status_Enum."Drive Motor") -> (w179:T10)
      }
      frame "Decelerate" {
        n154 = Unbundle By Name(w191) -> ("Y Data"=w190:T10)
        n155 = Unbundle By Name(w191) -> ("Timing.Loop time"=w194:dbl)
        n156 = Unbundle By Name(w190) -> ("SP.Speed"=w184:dbl, "Input.Decel"=w192:dbl)
        n157 = Multiply(x=w192, y=w194) -> (x*y=w187:dbl)
        n158 = Subtract(x=w184, y=w187) -> (x-y=w181:dbl)
        n159 = Less Than 0?(x=w181) -> (x < 0?=w185:bool)
        n160 = Select(t=0.0, s=w185, f=w181) -> (s? t:f=w183:dbl)
        n161 = Bundle By Name(cluster=w190, "Motor Params.Duty %"=0.5, "SP.Speed"=w183, "SP.Y Decel"=w187, "State"=Motor_Status_Enum."Drive Motor") -> (w189:T10)
      }
      frame "Drive Motor" {
        n162 = Unbundle By Name(w201) -> ("Y Data"=w198:T10)
        n163 = Unbundle By Name(w198) -> ("Motor Params.Freq"=w200:dbl, "Motor Params.FWD/RVS"=w199:bool, "Motor Params.Duty %"=w195:dbl)
        n164 = call "Y_axis_sub_VI.vi"("error in (no error)"=w203, "Duty Cycle"=w195, "FWD/RVS"=w199, "Frequency"=w200) -> ("error out"=w202:errorcluster)  [unwired: 7 in]
        n165 = Bundle By Name(cluster=w198, "State"=Motor_Status_Enum."Update I/O") -> (w197:T10)
      }
    }
    n166 = Bundle By Name(cluster=w79, "X Data"=w48, "Y Data"=w66) -> (w28:T1)
    n167 = Merge Errors(w67, w68) -> (w19:errorcluster)
    n168 = Unbundle By Name(w28) -> ("X Data.Motion.Dist"=w27:dbl, "X Data.SP.Speed"=w26:dbl, "X Data.Motion.Speed"=w25:dbl, "X Data.Motion.Acceleration"=w24:dbl, "Y Data.Motion.Dist"=w23:dbl, "Y Data.SP.Speed"=w22:dbl, "Y Data.Motion.Speed"=w21:dbl, "Y Data.Motion.Acceleration"=w20:dbl, "X Data.Complete?"=w15:bool, "Y Data.Complete?"=w14:bool)
    n169 = And(x=w15, y=w14) -> (x .and. y?=w16:bool)
    n170 = Bundle By Name(cluster=T6 {"X Axis"={"Displacement"=0.0, "Speed SP"=0.0, "Speed PV"=0.0, "Acceleration"=0.0}, "Y Axis"={"Displacement"=0.0, "Speed SP"=0.0, "Speed PV"=0.0, "Acceleration"=0.0}, "XY Complete?"=FALSE} ("XY Telemetry"), "X Axis.Displacement"=w27, "X Axis.Speed SP"=w26, "X Axis.Speed PV"=w25, "X Axis.Acceleration"=w24, "Y Axis.Displacement"=w23, "Y Axis.Speed SP"=w22, "Y Axis.Speed PV"=w21, "Y Axis.Acceleration"=w20, "XY Complete?"=w16) -> (w29:T6)
    n171 = shared-variable "NI-myRIO-1900-03050ae4\\Shared Variables.lvlib\\XY Telemetry"(w29, error in=w19) -> (error out=w18:errorcluster)
  }
  "XY Cluster Out" <- w5
  n172 = xnode "Y-axis PWM"("Duty Cycle"=w3, "Frequency [Hz]"=w3, "error in (no error)"=w2) -> ("error out"=w4:errorcluster)
  n173 = xnode "X-axis PWM"("Duty Cycle"=w3, "Frequency [Hz]"=w3, "error in (no error)"=w4) -> ("error out"=→"error out":errorcluster)
